vi "Read VIP_Path.vi"(8 "error in (no error)":errorcluster, 11 "VIPB Build in":refnum<class "VIP Publish.lvclass">) -> (0 "error out":errorcluster, 2 "VIPB_Path":path, 3 "VIPB Build out":refnum<class "VIP Publish.lvclass">)   [LabVIEW 2014, in "VIP Publish.lvclass"]
uses:
  VIP Publish.lvclass
  VIP Publish.lvclass/VIP Publish.ctl
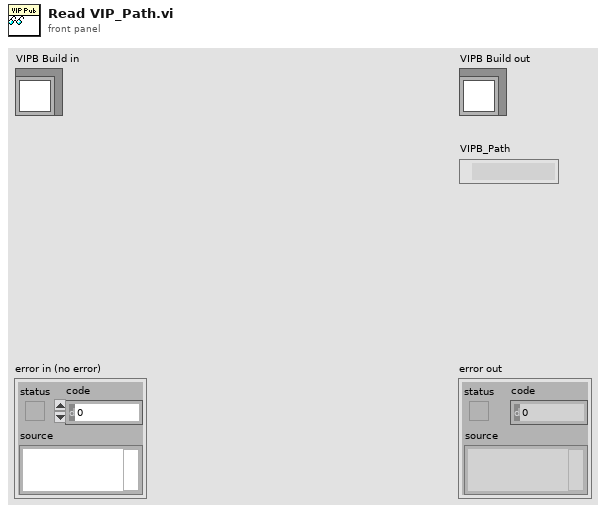
[diagram p1: front panel]
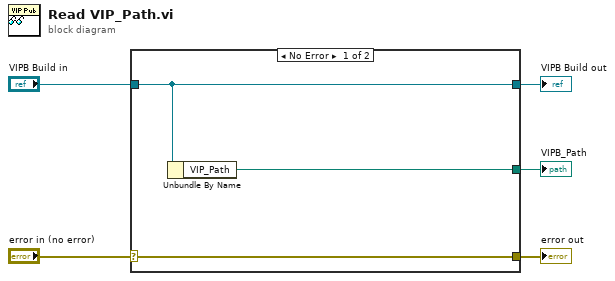
[diagram p0: block diagram]
diagram:
  n1 = case shown="No Error" "error in (no error)" {
    selector: "error in (no error)" -> [w8 w9]
    tunnel: [w8 w9] -> w4
    tunnel: [w7 w10] -> w2
    tunnel: "VIPB Build in" -> [w7 w10]
    tunnel: [w6 _] -> w1
    frame No Error {
      n2 = Unbundle By Name(w7) -> ("VIP_Path"=w6:path)
    }
    frame Error {
    }
  }
  "error out" <- w4
  "VIPB Build out" <- w2
  "VIPB_Path" <- w1
